vi "Set configuration chain.vi"(8 "error in (no error)":errorcluster, 9 "class names":string[](array[string]), 10 "configuration":variant[](array[variant]), 11 "waveform_FPGA in":refnum<class "waveform_FPGA.lvclass">) -> (0 "error out":errorcluster, 3 "waveform_FPGA out":refnum<class "waveform_FPGA.lvclass">)   [LabVIEW 2012, in "waveform_FPGA.lvclass"]
uses:
  waveform_FPGA.lvclass
  <vilib>/Distrio/Murmex/Murmex/Murmex.lvclass
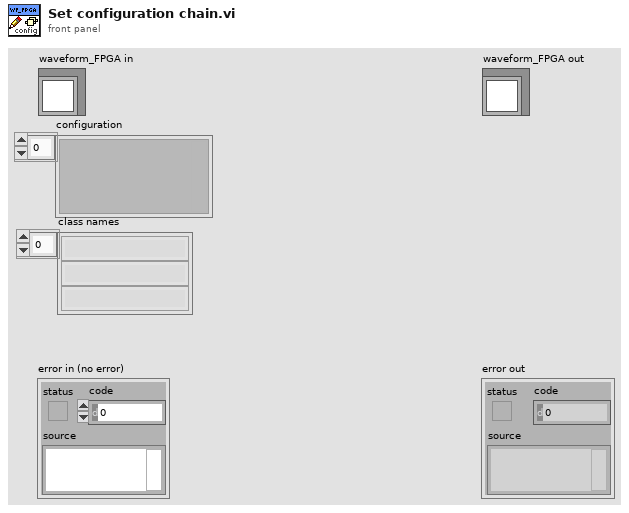
[diagram p1: front panel]
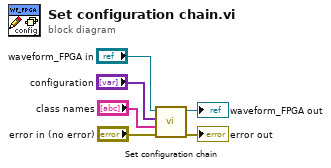
[diagram p0: block diagram]
diagram:
  n1 = call-parent "Set configuration chain.vi"("error in (no error)"="error in (no error)", "class names"="class names", "configuration"="configuration", "Murmex in"="waveform_FPGA in") -> ("error out"=→"error out":errorcluster, "Murmex out"=→"waveform_FPGA out":refnum<class "waveform_FPGA.lvclass">)  [unwired: 6 in]
